vi "ADIS16448 Loop.vi"(8 "error in":errorcluster) -> ()   [LabVIEW 2025]
uses:
  <vilib>/Rock Robotics/WPI/ThirdParty/ADI/ADIS16448/Typedef/ADIS16448 Device Reference.ctl
  <vilib>/Rock Robotics/WPI/ThirdParty/ADI/ADIS16448/Typedef/ADIS16448 Hardware Configuration.ctl
  <vilib>/Rock Robotics/WPI/SPI/WPI_SPIMode.ctl
  <vilib>/Rock Robotics/SystemInterfaces/DIO/FPGA_DIOChannel.ctl
  <vilib>/Rock Robotics/SystemInterfaces/spilib/spi_bus.ctl
  <vilib>/Rock Robotics/WPI/ThirdParty/ADI/ADIS16448/Typedef/ADIS16448 Status.ctl
  <vilib>/Rock Robotics/WPI/ThirdParty/ADI/ADIS16448/Typedef/ADIS16448 Process.ctl
  <vilib>/Rock Robotics/WPI/ThirdParty/ADI/ADIS16448/Typedef/ADIS16448 Command Type.ctl
  <vilib>/Rock Robotics/SystemInterfaces/CounterEncoderSourceConvertion/FPGA_CounterEncoderSourceConvertionLVSourceType.ctl
  <vilib>/Rock Robotics/SystemInterfaces/DIO/FPGA_DIODigitalSourceChannel.ctl
  <vilib>/Rock Robotics/SystemInterfaces/AnalogTrigger/FPGA_AnalogTriggerIndex.ctl
  <vilib>/Rock Robotics/SystemInterfaces/AnalogTrigger/FPGA_AnalogTriggerOutType.ctl
  <vilib>/Rock Robotics/WPI/ThirdParty/ADI/ADIS16448/Typedef/ADIS16448 Data.ctl
  <vilib>/Rock Robotics/WPI/SPI/WPI_SPIDevRef.ctl
  <vilib>/Rock Robotics/WPI/ThirdParty/ADI/ADIS16448/Typedef/ADIS16448 Register.ctl
  <vilib>/Rock Robotics/WPI/Counter/WPI_CounterDigitalInputToDigitalSource.vi
panel:
  in  "ADIS16448DevRef":T1={"DevStatus"={"status"=FALSE, "code"=0, "source"=""}, "Hardware Config"={"SPI Clock Rate (Hz)"=1000000.0, "IMU SPI Mode (3)"=enum."Mode 3 (Clk Idle High,Sample on Trailing)", "IMU Reset Pin"=enum."SPI Port CS2", "IMU SPI Bus"=enum."SPI On-Board, CS0", "IMU Data Ready Pin"=enum."SPI Port CS1", "Stall Config"={"Pow2BytesPerRead"=255, "StallTicks"=640, "CsToSclkTicks"=5}, "IMU Status LED Pin"=enum."DIO MXP 9"}, "Calibration Complete"=refnum, "Status reference"=refnum, "Sychronous Process VI"=refnum, "Cmd FIFO"=refnum, "Source"={"DevStatus"={"status"=FALSE, "code"=0, "source"=""}, "AnalogTriggerMode?"=FALSE, "DigitalMode"={"DIO Channel"=enum."Disabled"}, "AnalogTriggerMode"={"AnalogTriggerIndex"=enum."Trig 0", "OutputType"=enum."InWindow"}}, "Data FIFO"=refnum, "IMU Status LED Pin"=enum."DIO MXP 9", "Calibration Time (ms)"=5, "Data Reference"=refnum}
  in  "Main Name":string
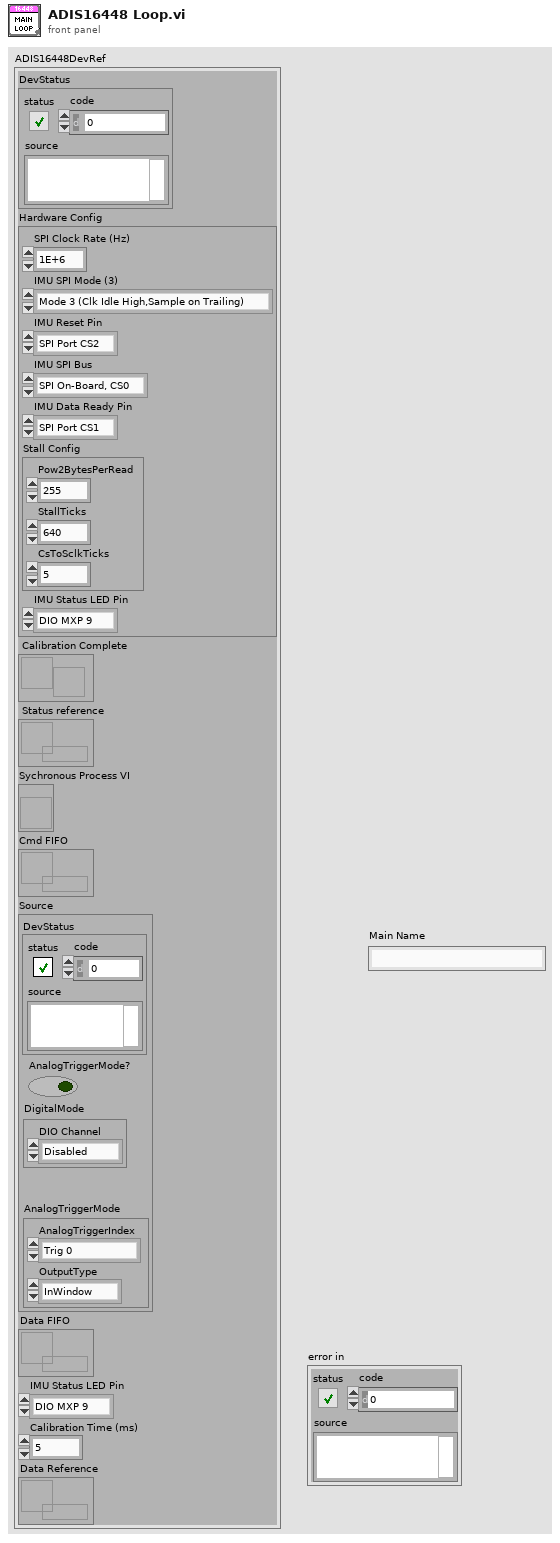
[diagram p1: front panel]
types:
  T1 = typedef "ADIS16448 Device Reference.ctl" = cluster{"DevStatus":errorcluster, "Hardware Config":T2, "Calibration Complete":refnum<notifier>, "Status reference":refnum<data-value>, "Sychronous Process VI":T6, "Cmd FIFO":refnum<k33>, "Source":T7, "Data FIFO":refnum<k33>, "IMU Status LED Pin":T4, "Calibration Time (ms)":u32, "Data Reference":refnum<data-value>}
  T2 = typedef "ADIS16448 Hardware Configuration.ctl" = cluster{"SPI Clock Rate (Hz)":dbl, "IMU SPI Mode (3)":T3, "IMU Reset Pin":T4, "IMU SPI Bus":T5, "IMU Data Ready Pin":T4, "Stall Config":cluster{"Pow2BytesPerRead":u8, "StallTicks":u16, "CsToSclkTicks":u8}, "IMU Status LED Pin":T4}
  T3 = typedef "WPI_SPIMode.ctl" = enum16{"Mode 0 (Clk Idle Low,Sample on Leading)", "Mode 1 (Clk Idle Low,Sample on Trailing)", "Mode 2 (Clk Idle High,Sample on Leading)", "Mode 3 (Clk Idle High,Sample on Trailing)"}
  T4 = typedef "FPGA_DIOChannel.ctl" = enum8{"DIO 0", "DIO 1", "DIO 2", "DIO 3", "DIO 4", "DIO 5", "DIO 6", "DIO 7", "DIO 8", "DIO 9", "DIO MXP 0", "DIO MXP 1", "DIO MXP 2", "DIO MXP 3", "DIO MXP 4", "DIO MXP 5", "DIO MXP 6", "DIO MXP 7", "DIO MXP 8", "DIO MXP 9", "DIO MXP 10", "DIO MXP 11", "DIO MXP 12", "DIO MXP 13", "DIO MXP 14", "DIO MXP 15", "SPI Port CS1", "SPI Port CS2", "SPI Port CS3", "SPI Port MISO", "SPI Port MOSI", "Invalid"}
  T5 = typedef "spi_bus.ctl" = enum16{"SPI On-Board, CS0", "SPI On-Board, CS1", "SPI On-Board, CS2", "SPI On-Board, CS3", "SPI MXP", "Invalid"}
  T6 = typedef "ADIS16448 Process.ctl" = refnum<vi>
  T7 = typedef "FPGA_CounterEncoderSourceConvertionLVSourceType.ctl" = cluster{"DevStatus":errorcluster, "AnalogTriggerMode?":bool, "DigitalMode":cluster{"DIO Channel":T8}, "AnalogTriggerMode":cluster{"AnalogTriggerIndex":T9, "OutputType":T10}}
  T8 = typedef "FPGA_DIODigitalSourceChannel.ctl" = enum8{"DIO 0", "DIO 1", "DIO 2", "DIO 3", "DIO 4", "DIO 5", "DIO 6", "DIO 7", "DIO 8", "DIO 9", "DIO MXP 0", "DIO MXP 1", "DIO MXP 2", "DIO MXP 3", "DIO MXP 4", "DIO MXP 5", "DIO MXP 6", "DIO MXP 7", "DIO MXP 8", "DIO MXP 9", "DIO MXP 10", "DIO MXP 11", "DIO MXP 12", "DIO MXP 13", "DIO MXP 14", "DIO MXP 15", "SPI Port CS1", "SPI Port CS2", "SPI Port CS3", "SPI Port MISO", "SPI Port MOSI", "Disabled"}
  T9 = typedef "FPGA_AnalogTriggerIndex.ctl" = enum8{"Trig 0", "Trig 1", "Trig 2", "Trig 3", "Trig 4", "Trig 5", "Trig 6", "Trig 7", "Invalid"}
  T10 = typedef "FPGA_AnalogTriggerOutType.ctl" = enum16{"InWindow", "TriggerState", "Rising", "Falling"}
  T11 = typedef "WPI_SPIDevRef.ctl" = cluster{"DevStatus":errorcluster, "Handle":i32, "SPI Bus":T5}
  T12 = typedef "ADIS16448 Data.ctl" = cluster{"XAngle":dbl, "YAngle":dbl, "ZAngle":dbl}
  T13 = cluster{"SPIDevRef":T11, "Data Counter":u16, "Digital Source":T7, "Bytes Per Sample":u32, "Data":T12, "ADIS16448DevRef":T1, "TimeStampPrev":u32, "Sensor to Robot Rotation":dbl[][], "AutoSPI Active?":bool, "Offsets":T12, "Data Header":u8[], "Zero Byte Count":u8, "Reset":bool}
  T14 = typedef "ADIS16448 Status.ctl" = cluster{"Calibrated?":bool, "IMU Detected?":bool}
  T15 = typedef "ADIS16448 Register.ctl" = u8
  T16 = typedef "ADIS16448 Command Type.ctl" = cluster{"Command":enum16{"None", "Reset", "Recalibrate"}, "Data":u32}
  T17 = typedef "WPI_DigitalOutputDevRef.ctl" = cluster{"DIO Channel":T4, "DevStatus":errorcluster}
  T18 = typedef "WPI_DigitalInputDevRef.ctl" = cluster{"DevStatus":errorcluster, "DIO Channel":T4}
  T19 = cluster{"Pow2BytesPerRead":u8, "StallTicks":u16, "CsToSclkTicks":u8}
  T20 = enum32{"Bad", "Idle", "Run top level", "Running"}
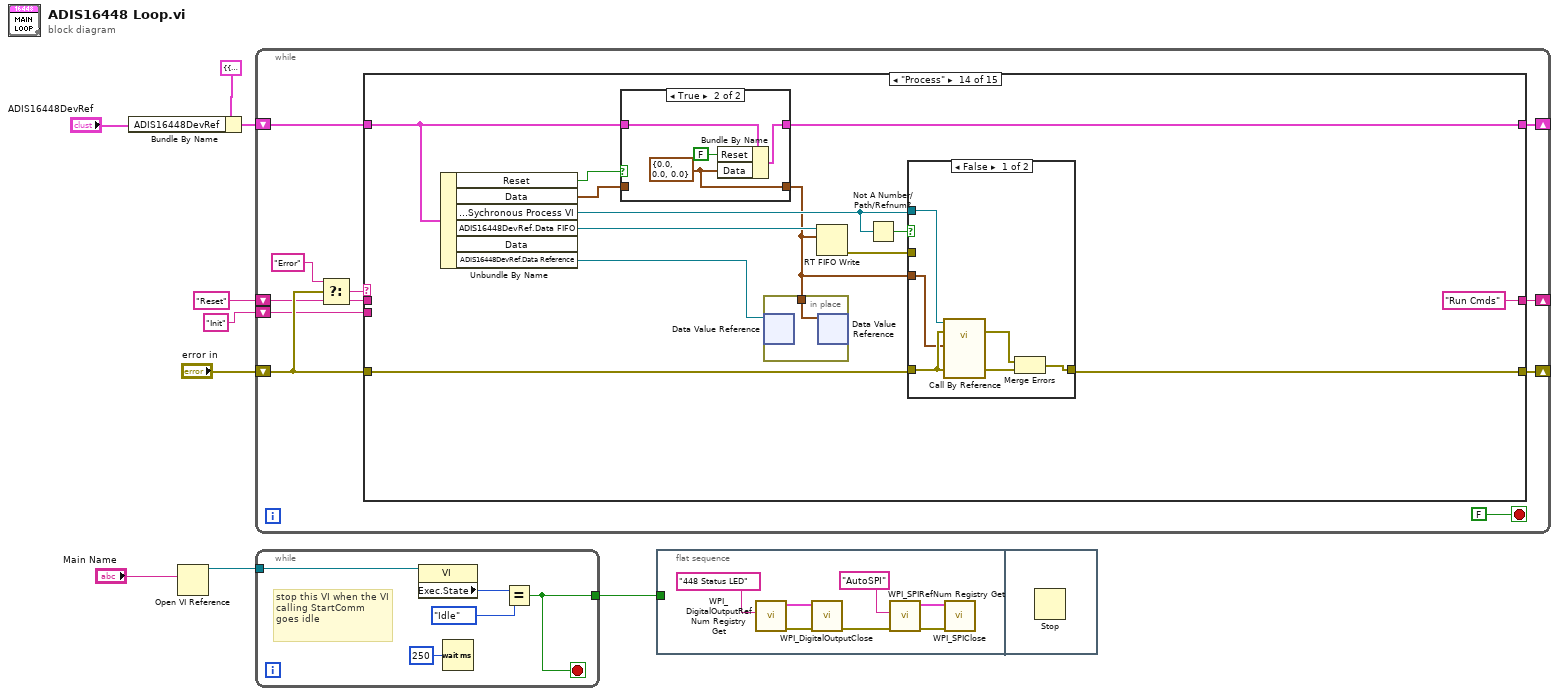
[diagram p0: block diagram]
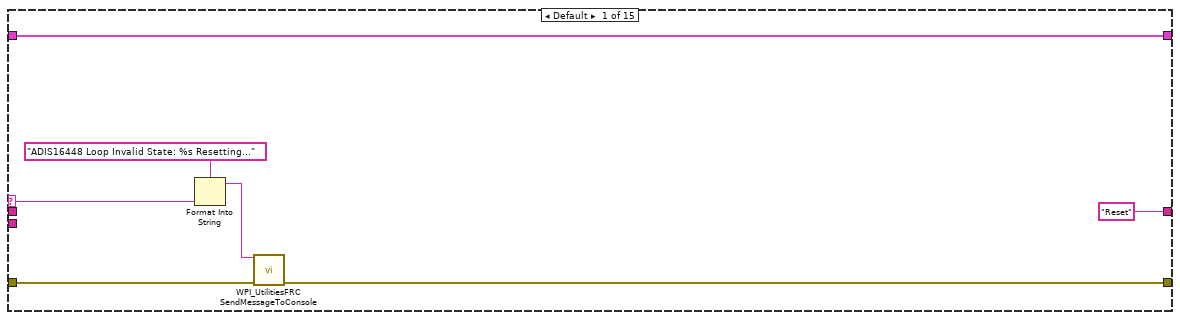
[diagram p2: hidden frame]
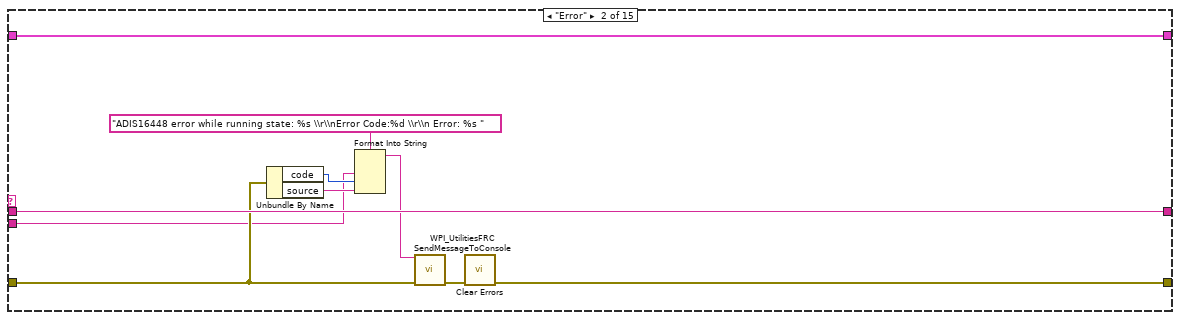
[diagram p3: hidden frame]
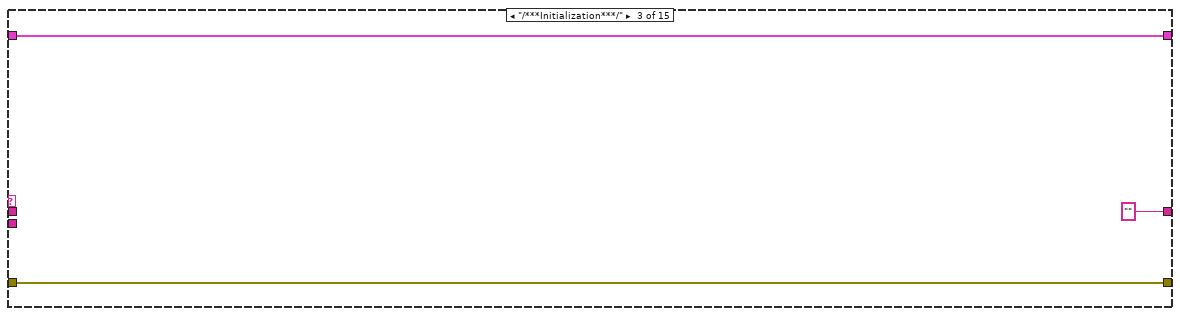
[diagram p4: hidden frame]
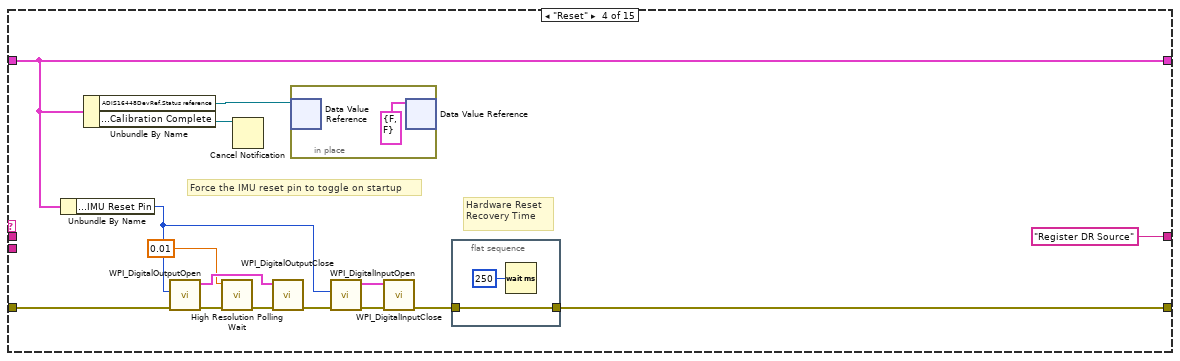
[diagram p5: hidden frame]
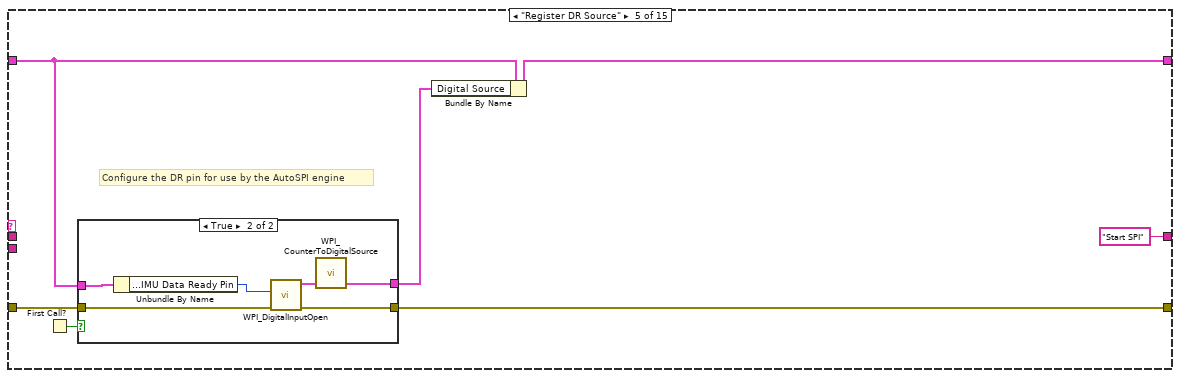
[diagram p6: hidden frame]
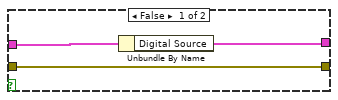
[diagram p7: hidden frame]
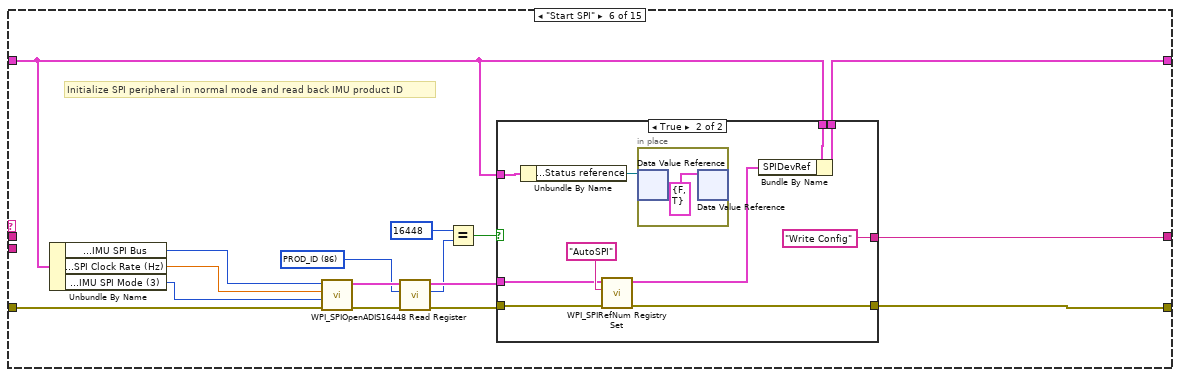
[diagram p8: hidden frame]
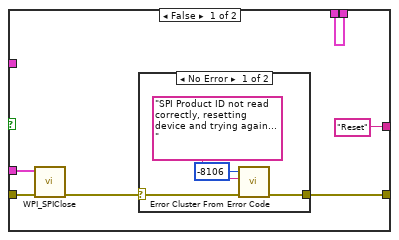
[diagram p9: hidden frame]
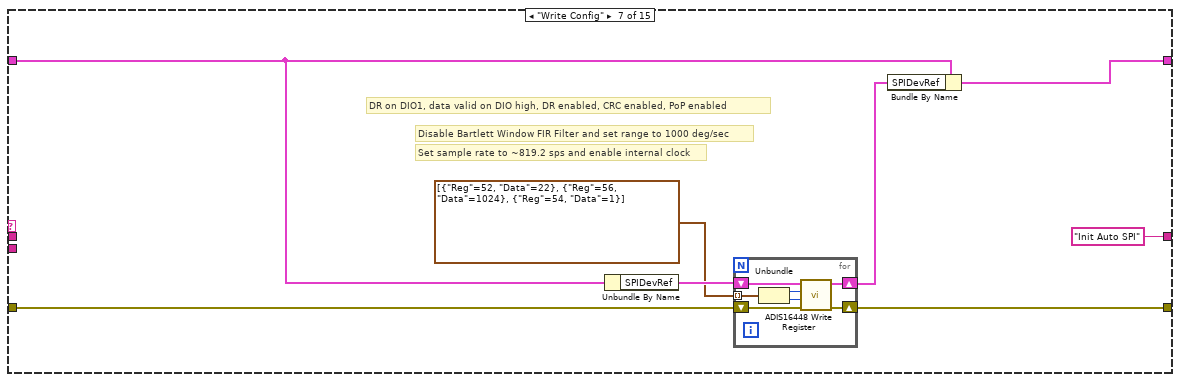
[diagram p11: hidden frame]
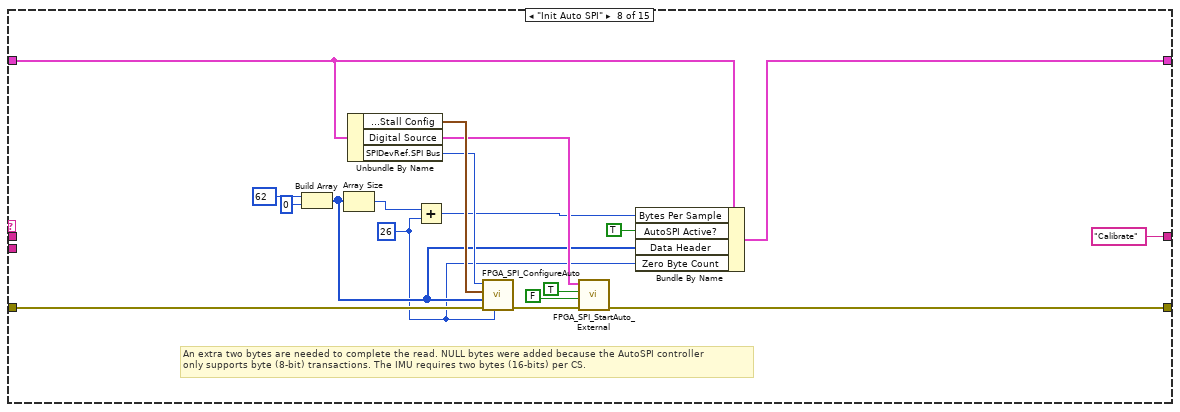
[diagram p12: hidden frame]
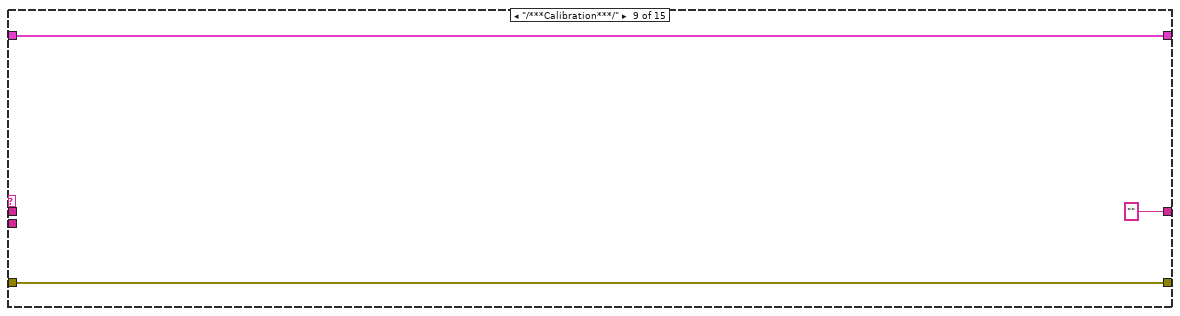
[diagram p13: hidden frame]
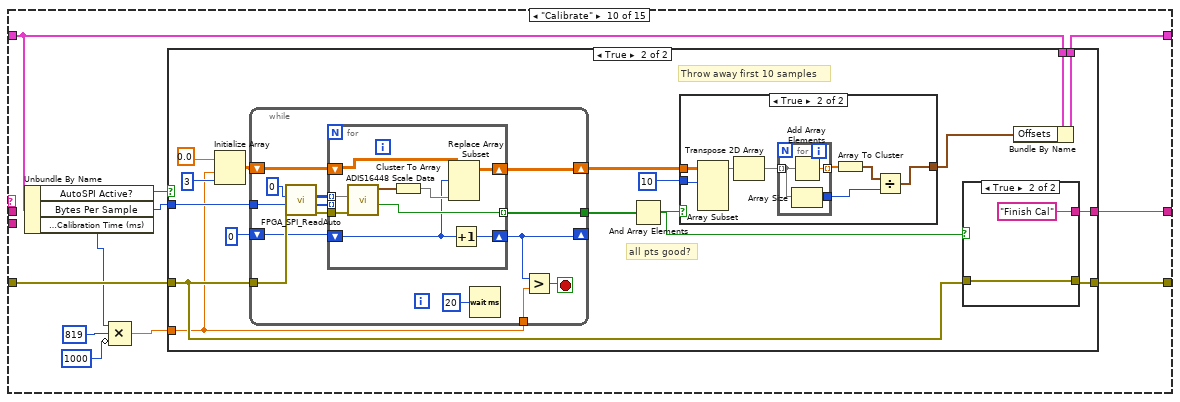
[diagram p14: hidden frame]
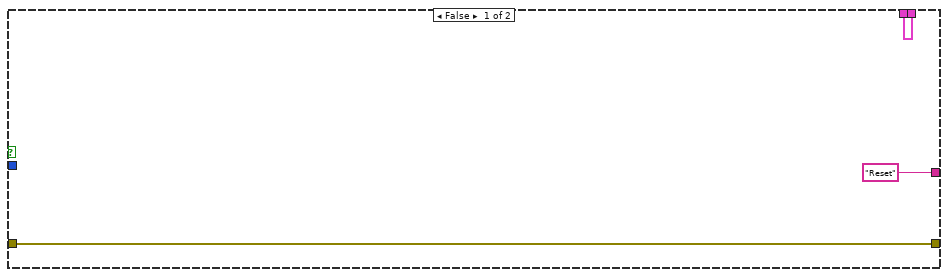
[diagram p15: hidden frame]
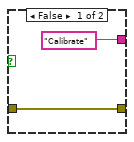
[diagram p17: hidden frame]
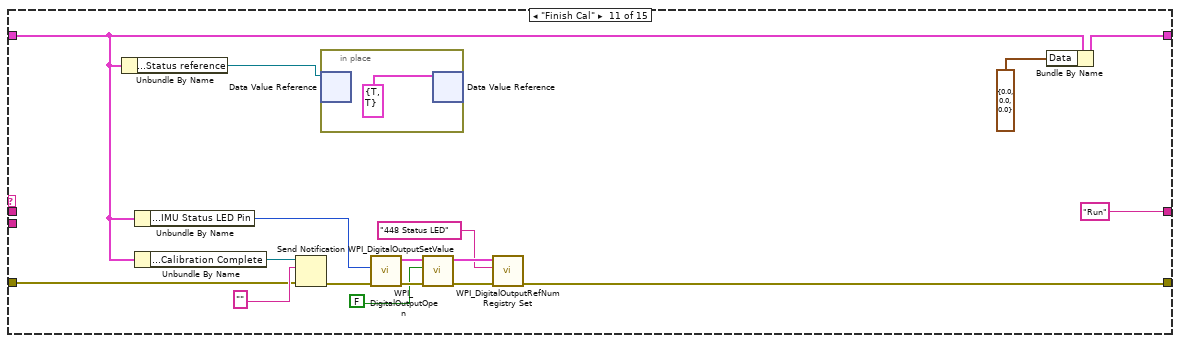
[diagram p18: hidden frame]
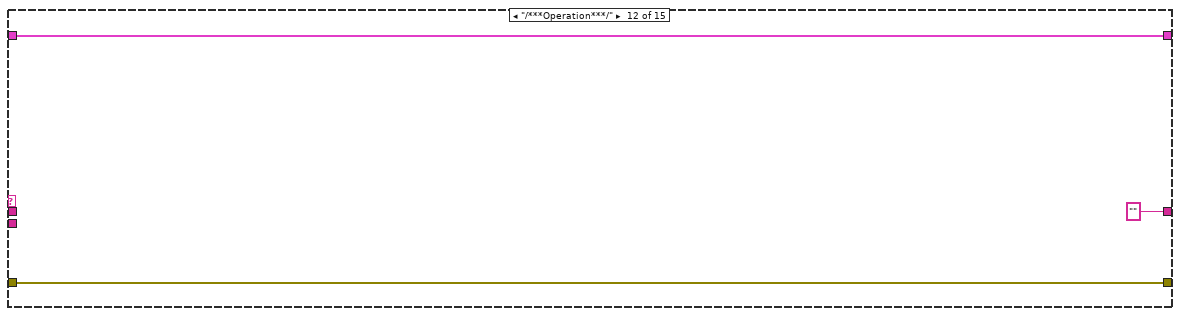
[diagram p19: hidden frame]
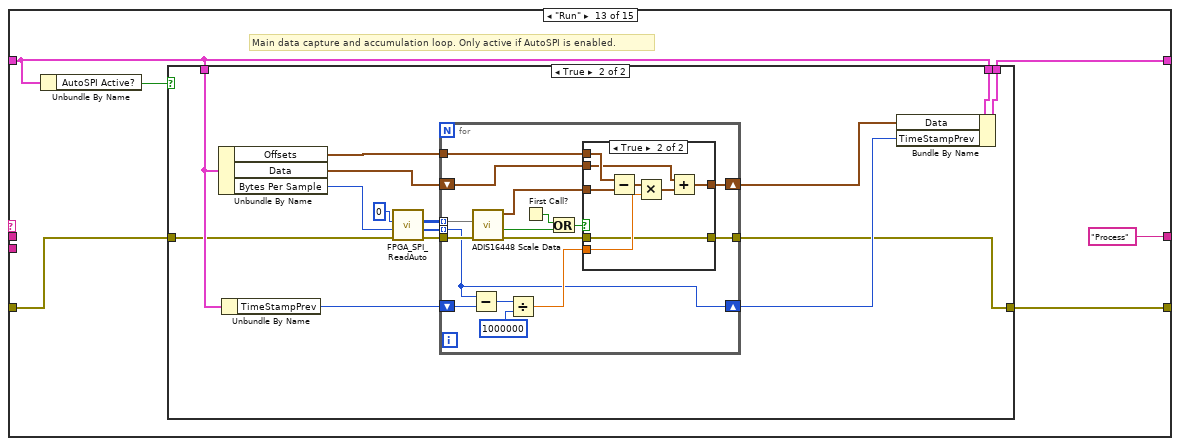
[diagram p20: hidden frame]
diagram:
  n1 = Bundle By Name(cluster=T13 {"SPIDevRef"={"DevStatus"={"status"=FALSE, "code"=0, "source"=""}, "Handle"=0, "SPI Bus"=enum."SPI On-Board, CS0"}, "Data Counter"=0, "Digital Source"={"DevStatus"={"status"=FALSE, "code"=0, "source"=""}, "AnalogTriggerMode?"=FALSE, "DigitalMode"={"DIO Channel"=enum."DIO 1"}, "AnalogTriggerMode"={"AnalogTriggerIndex"=enum."Trig 0", "OutputType"=enum."InWindow"}}, "Bytes Per Sample"=0, "Data"={"XAngle"=0.0, "YAngle"=0.0, "ZAngle"=0.0}, "ADIS16448DevRef"={"DevStatus"={"status"=FALSE, "code"=0, "source"=""}, "Hardware Config"={"SPI Clock Rate (Hz)"=1000000.0, "IMU SPI Mode (3)"=enum."Mode 3 (Clk Idle High,Sample on Trailing)", "IMU Reset Pin"=enum."SPI Port CS2", "IMU SPI Bus"=enum."SPI On-Board, CS0", "IMU Data Ready Pin"=enum."SPI Port CS1", "Stall Config"={"Pow2BytesPerRead"=255, "StallTicks"=640, "CsToSclkTicks"=5}, "IMU Status LED Pin"=enum."DIO MXP 9"}, "Calibration Complete"=refnum, "Status reference"=refnum, "Sychronous Process VI"=refnum, "Cmd FIFO"=refnum, "Source"={"DevStatus"={"status"=FALSE, "code"=0, "source"=""}, "AnalogTriggerMode?"=FALSE, "DigitalMode"={"DIO Channel"=enum."Disabled"}, "AnalogTriggerMode"={"AnalogTriggerIndex"=enum."Trig 0", "OutputType"=enum."InWindow"}}, "Data FIFO"=refnum, "IMU Status LED Pin"=enum."DIO MXP 9", "Calibration Time (ms)"=5, "Data Reference"=refnum}, "TimeStampPrev"=0, "Sensor to Robot Rotation"=[], "AutoSPI Active?"=TRUE, "Offsets"={"XAngle"=0.0, "YAngle"=0.0, "ZAngle"=0.0}, "Data Header"=[], "Zero Byte Count"=0, "Reset"=TRUE}, "ADIS16448DevRef"="ADIS16448DevRef") -> (w5:T13)
  n2 = Open VI Reference(vi path="Main Name") -> (vi reference=w8:refnum<vi>)  [unwired: 3 in, 3 out]
  n3 = while {
    shift-right: [w15] -> _
    shift-left: "Reset" -> [w12]
    shift-right: [w17] -> _
    shift-left: w5 -> [w18]
    shift-right: [w16] -> _
    shift-left: "error in" -> [w14]
    shift-left: "Init" -> [w10]
    stop <- FALSE stop-if-true
    n4 = Select(t="Error", s=w14, f=w12) -> (s? t:f=w13:string)
    n5 = case shown="\"Process\"" w13 {
      selector: w13 -> [w25 _ _ _ _ _ _ _ _ _ _ _ _ _ _]
      tunnel: w18 -> [w26 w36 w39 w40 w59 w78 w114 w139 w147 w152 w227 w236 w238 w289 w316]
      tunnel: [w26 w36 w39 w40 w63 w83 w113 w138 w147 w155 w231 w236 w241 w290 w322] -> w17
      tunnel: w14 -> [w24 w32 w38 w46 w62 w89 w117 w143 w146 w157 w228 w235 w240 w296 w324]
      tunnel: [w23 w33 w38 w53 w60 w82 w116 w127 w146 w156 w220 w235 w239 w295 w323] -> w16
      tunnel: ["Reset" w35 "" "Register DR Source" "Start SPI" w84 "Init Auto SPI" "Calibrate" "" w153 "Run" "" "Process" "Run Cmds" w314] -> w15
      tunnel: w12 -> [_ w35 _ _ _ _ _ _ _ _ _ _ _ _ _]
      tunnel: w10 -> [_ w27 _ _ _ _ _ _ _ _ _ _ _ _ _]
      frame Default {
        n6 = Format Into String(format string="ADIS16448 Loop Invalid State: %s Resetting...", w25) -> (resulting string=w22:string)  [unwired: 2 in, 1 out]
        n7 = call <vilib>:"WPI_UtilitiesFRC SendMessageToConsole.vi"("Message"=w22, "error in (no error)"=w24) -> ("error out"=w23:errorcluster)  [unwired: 13 in]
      }
      frame "Error" {
        n8 = Unbundle By Name(w32) -> ("code"=w29:i32, "source"=w28:string)
        n9 = Format Into String(format string="ADIS16448 error while running state: %s \\r\\nError Code:%d \\r\\n Error: %s ", w27, w29, w28) -> (resulting string=w31:string)  [unwired: 2 in, 1 out]
        n10 = call <vilib>:"WPI_UtilitiesFRC SendMessageToConsole.vi"("Message"=w31, "error in (no error)"=w32) -> ("error out"=w34:errorcluster)  [unwired: 13 in]
        n11 = call <vilib>:"Clear Errors.vi"("error in (no error)"=w34) -> ("error out"=w33:errorcluster)  [unwired: 5 in, 1 out]
      }
      frame "/***Initialization***/" {
      }
      frame "Reset" {
        # "Hardware Reset Recovery Time"
        # "Force the IMU reset pin to toggle on startup"
        n12 = Unbundle By Name(w40) -> ("ADIS16448DevRef.Hardware Config.IMU Reset Pin"=w42:T4)
        n13 = Unbundle By Name(w40) -> ("ADIS16448DevRef.Status reference"=w41:refnum<data-value>, "ADIS16448DevRef.Calibration Complete"=w52:refnum<notifier>)
        n14 = call <vilib>:"WPI_DigitalOutputOpen.vi"("error in (no error)"=w46, "DIO Channel"=w42) -> ("error out"=w44:errorcluster, "DigitalOutputDevRef"=w51:T17)  [unwired: 8 in]
        n15 = call <vilib>:"High Resolution Polling Wait.vi"("error in (no error)"=w44, "seconds to wait"=0.01) -> ("error out"=w45:errorcluster)  [unwired: 9 in]
        n16 = Cancel Notification(0:w52) -> ()  [unwired: 1 in, 3 out]
        n17 = call <vilib>:"WPI_DigitalOutputClose.vi"("error in (no error)"=w45, "DigitalOutputDevRef"=w51) -> ("error out"=w48:errorcluster)  [unwired: 9 in]
        n18 = in-place {
          n19 = in-place-dvr #1(w41) -> ()  [unwired: 2 out]
          n20 = in-place-dvr #1(T14 {"Calibrated?"=FALSE, "IMU Detected?"=FALSE} ("element")) -> ()  [unwired: 2 out]
        }
        n21 = call <vilib>:"WPI_DigitalInputOpen.vi"("error in (no error)"=w48, "DIO Channel"=w42) -> ("error out"=w49:errorcluster, "DigitalInputDevRef"=w50:T18)  [unwired: 8 in]
        n22 = call <vilib>:"WPI_DigitalInputClose.vi"("error in (no error)"=w49, "DigitalInputDevRef"=w50) -> ("error out"=w47:errorcluster)  [unwired: 9 in]
        n23 = flat-sequence {
          tunnel: [w57] -> w53
          tunnel: w47 -> [w57]
          frame #0 {
            n24 = Wait (ms)(milliseconds to wait=u32 250) -> ()  [unwired: 1 out]
          }
        }
      }
      frame "Register DR Source" {
        # "Configure the DR pin for use by the AutoSPI engine"
        n25 = First Call?() -> (First Call?: T/F=w58:bool)
        n26 = case shown="True" w58 {
          tunnel: w62 -> [w65 w73]
          tunnel: w59 -> [w67 w71]
          tunnel: [w66 w69] -> w61
          tunnel: [w65 w68] -> w60
          frame False {
            n27 = Unbundle By Name(w67) -> ("Digital Source"=w66:T7)
          }
          frame True {
            n28 = Unbundle By Name(w71) -> ("ADIS16448DevRef.Hardware Config.IMU Data Ready Pin"=w70:T4)
            n29 = call <vilib>:"WPI_DigitalInputOpen.vi"("error in (no error)"=w73, "DIO Channel"=w70) -> ("error out"=w68:errorcluster, "DigitalInputDevRef"=w72:T18)  [unwired: 8 in]
            n30 = call-poly <vilib>:"WPI_CounterToDigitalSource.vi"("DigitalInputDevRef"=w72) -> ("Digital Source"=w69:T7)  [unwired: 6 in]
          }
        }
        n31 = Bundle By Name(cluster=w59, "Digital Source"=w61) -> (w63:T13)
      }
      frame "Start SPI" {
        w77 = T15 86 items=["FLASH_CNT"=0, "Reserved 1"=2, "XGYRO_OUT"=4, "YGYRO_OUT"=6, "ZGYRO_OUT"=8, "XACCL_OUT"=10, "YACCL_OUT"=12, "ZACCL_OUT"=14, "XMAGN_OUT"=16, "YMAGN_OUT"=18, "ZMAGN_OUT"=20, "BARO_OUT"=22, "TEMP_OUT"=24, "XGYRO_OFF"=26, "YGYRO_OFF"=28, "ZGYRO_OFF"=30, "XACCL_OFF"=32, "YACCL_OFF"=34, "ZACCL_OFF"=36, "XMAGN_HIC"=38, "YMAGN_HIC"=40, "ZMAGN_HIC"=42, "XMAGN_SIC"=44, "YMAGN_SIC"=46, "ZMAGN_SIC"=48, "GPIO_CTRL"=50, "MSC_CTRL"=52, "SMPL_PRD"=54, "SENS_AVG"=56, "SEQ_CNT"=58, "DIAG_STAT"=60, "GLOB_CMD"=62, "ALM_MAG1"=64, "ALM_MAG2"=66, "ALM_SMPL1"=68, "ALM_SMPL2"=70, "ALM_CTRL"=72, "Reserved 2"=74, "Reserved 3"=76, "Reserved 4"=78, "Reserved 5"=80, "LOT_ID1"=82, "LOT_ID2"=84, "PROD_ID"=86, "SERIAL_NUM"=88] ("ADIS16448 Register")
        # "Initialize SPI peripheral in normal mode and read back IMU product ID"
        n32 = Unbundle By Name(w78) -> ("ADIS16448DevRef.Hardware Config.IMU SPI Bus"=w85:T5, "ADIS16448DevRef.Hardware Config.SPI Clock Rate (Hz)"=w86:dbl, "ADIS16448DevRef.Hardware Config.IMU SPI Mode (3)"=w87:T3)
        n33 = call <vilib>:"WPI_SPIOpen.vi"("error in"=w89, "Mode (3)"=w87, "Clock Rate (Hz)"=w86, "SPI Bus"=w85) -> ("error out"=w81:errorcluster, "SPIDevRef"=w80:T11)  [unwired: 6 in]
        n34 = call <vilib>:"ADIS16448 Read Register.vi"("error in (no error)"=w81, "ADIS16448 Register"=w77, "SPIDevRef in"=w80) -> ("error out"=w75:errorcluster, "Register Value"=w74:u16, "SPIDevRef out"=w76:T11)  [unwired: 6 in]
        n35 = Equal?(x=u16 16448 ("y"), y=w74) -> (x = y?=w88:bool)
        n36 = case shown="True" w88 {
          tunnel: ["Reset" "Write Config"] -> w84
          tunnel: w78 -> [w94 w109]
          tunnel: [w94 w108] -> w83
          tunnel: [w93 w103] -> w82
          tunnel: w75 -> [w92 w104]
          tunnel: w76 -> [w91 w105]
          tunnel: w78 -> [_ w102]
          frame False {
            n37 = call <vilib>:"WPI_SPIClose.vi"("error in (no error)"=w92, "SPIDevRef"=w91) -> ("error out"=w90:errorcluster)  [unwired: 9 in]
            n38 = case shown="No Error" w90 {
              selector: w90 -> [w98 w100]
              tunnel: [w99 w100] -> w93
              frame No Error {
                n39 = call <vilib>:"Error Cluster From Error Code.vi"("error in (no error)"=w98, "error message (\"\")"="SPI Product ID not read correctly, resetting device and trying again..." ("error message (\"\")"), "error code (0)"=-8106) -> ("error out"=w99:errorcluster)  [unwired: 6 in]
              }
              frame Error {
              }
            }
          }
          frame True {
            n40 = Unbundle By Name(w102) -> ("ADIS16448DevRef.Status reference"=w101:refnum<data-value>)
            n41 = call <vilib>:"WPI_SPIRefNum Registry Set.vi"("error in (no error)"=w104, "refnum name"="AutoSPI", "SPIDevRef"=w105) -> ("error out"=w103:errorcluster, "SPIDevRef"=w107:T11)  [unwired: 7 in]
            n42 = in-place {
              n43 = in-place-dvr #2(w101) -> ()  [unwired: 2 out]
              n44 = in-place-dvr #2(T14 {"Calibrated?"=FALSE, "IMU Detected?"=TRUE} ("element")) -> ()  [unwired: 2 out]
            }
            n45 = Bundle By Name(cluster=w109, "SPIDevRef"=w107) -> (w108:T13)
          }
        }
      }
      frame "Write Config" {
        # "DR on DIO1, data valid on DIO high, DR enabled, CRC enabled, PoP enabled"
        # "Set sample rate to ~819.2 sps and enable internal clock"
        # "Disable Bartlett Window FIR Filter and set range to 1000 deg/sec"
        n46 = Unbundle By Name(w114) -> ("SPIDevRef"=w118:T11)
        n47 = for {
          tunnel: cluster{"Reg":T15, "Data":u16}[] [{"Reg"=52, "Data"=22}, {"Reg"=56, "Data"=1024}, {"Reg"=54, "Data"=1}] -> [w126] mode=indexing
          shift-right: [w122] -> w116
          shift-left: w117 -> [w121]
          shift-right: [w120] -> w112
          shift-left: w118 -> [w123]
          n48 = Unbundle(w126) -> ("Reg"=w125:T15, "Data"=w124:u16)
          n49 = call <vilib>:"ADIS16448 Write Register.vi"("error in (no error)"=w121, "Data"=w124, "Register"=w125, "SPIDevRef in"=w123) -> ("error out"=w122:errorcluster, "SPIDevRef out"=w120:T11)  [unwired: 6 in]
        }
        n50 = Bundle By Name(cluster=w114, "SPIDevRef"=w112) -> (w113:T13)
      }
      frame "Init Auto SPI" {
        w128 = u8 26 ("dimension size")
        # "An extra two bytes are needed to complete the read. NULL bytes were added because the AutoSPI controller \nonly supports byte (8-bit) transactions. The IMU requires two bytes (16-bits) per CS."
        n51 = Build Array(u8 62 ("hi"), u8 0 ("element")) -> (w129:u8[])
        n52 = Array Size(array=w129) -> (size(s)=w133:i32)
        n53 = Unbundle By Name(w139) -> ("ADIS16448DevRef.Hardware Config.Stall Config"=w137:T19, "Digital Source"=w135:T7, "SPIDevRef.SPI Bus"=w134:T5)
        n54 = Add(x=w133, y=w128) -> (x+y=w130:i32)
        n55 = call <vilib>:"FPGA_SPI_ConfigureAuto.vi"("SPI Auto Zero Byte Count"=w128, "error in"=w143, "SPI Auto TX Byte Array"=w129, "Stall Config"=w137, "SPI Bus"=w134) -> ("error out"=w142:errorcluster)  [unwired: 6 in]
        n56 = call <vilib>:"FPGA_SPI_StartAuto_External.vi"("error in (no error)"=w142, "Falling Edge"=FALSE, "Rising Edge"=TRUE, "Source"=w135) -> ("error out"=w127:errorcluster)  [unwired: 7 in]
        n57 = Bundle By Name(cluster=w139, "Bytes Per Sample"=w130, "AutoSPI Active?"=TRUE, "Data Header"=w129, "Zero Byte Count"=w128) -> (w138:T13)
      }
      frame "/***Calibration***/" {
      }
      frame "Calibrate" {
        n58 = Unbundle By Name(w152) -> ("AutoSPI Active?"=w158:bool, "Bytes Per Sample"=w154:u32, "ADIS16448DevRef.Calibration Time (ms)"=w150:u32)
        n59 = Compound Arithmetic op=MULTIPLY(w150, 819, invert 1000) -> (w149:dbl)
        n60 = case shown="True" w158 {
          tunnel: [w161 w177] -> w155
          tunnel: w157 -> [w160 w165]
          tunnel: [w160 w173] -> w156
          tunnel: w152 -> [w161 w176]
          tunnel: w154 -> [_ w175]
          tunnel: ["Reset" w174] -> w153
          tunnel: w149 -> [_ w163]
          frame False {
          }
          frame True {
            # "all pts good?"
            # "Throw away first 10 samples"
            n61 = Initialize Array(0.0, w163, 3) -> (w167:dbl[][])
            n62 = while {
              tunnel: w175 -> [w187]
              tunnel: w165 -> [w186]
              tunnel: [w185] -> w172
              tunnel: w163 -> [w179]
              shift-right: [w182] -> w164
              shift-left: w167 -> [w183]
              shift-right: [w180] -> _
              shift-left: u32 0 ("Samples to Read") -> [w181]
              stop <- w178 stop-if-true
              n63 = call <vilib>:"FPGA_SPI_ReadAuto.vi"("error in (no error)"=w186, "Bytes per Sample"=w187, "Samples to Read"=u32 0) -> ("error out"=w188:errorcluster, "Timestamps"=w189:u32[], "Data"=w190:u8[][])  [unwired: 6 in]
              n64 = for {
                tunnel: w190 -> [w200] mode=indexing
                tunnel: w189 -> [_] mode=indexing
                tunnel: w188 -> [w199]
                tunnel: [w198] -> w185 mode=indexing
                shift-right: [w195] -> w182
                shift-left: w183 -> [w196]
                shift-right: [w197] -> w180
                shift-left: w181 -> [w193]
                n65 = call <vilib>:"ADIS16448 Scale Data.vi"("error in (no error)"=w199, "New Data In"=w200) -> ("Data Good?"=w198:bool, "output cluster"=w192:T12)  [unwired: 6 in, 2 out]
                n66 = Cluster To Array(cluster=w192) -> (array=w194:dbl[])
                n67 = Replace Array Subset(array=w196, new element=w194, index (row)=w193) -> (w195:dbl[][])  [unwired: 1 in]
                n68 = Increment(x=w193) -> (x+1=w197:u32)
              }
              n69 = Wait (ms)(milliseconds to wait=u32 20) -> ()  [unwired: 1 out]
              n70 = Greater?(x=w180, y=w179) -> (0:w178:bool)
            }
            n71 = And Array Elements(Boolean array=w172) -> (logical AND=w170:bool)
            n72 = case shown="True" w170 {
              tunnel: 10 -> [_ w207]
              tunnel: w164 -> [_ w208]
              tunnel: [_ w203] -> w162
              frame False {
              }
              frame True {
                n73 = Array Subset(array=w208, index (row)=w207) -> (w206:dbl[][])  [unwired: 3 in]
                n74 = Transpose 2D Array(2D array=w206) -> (transposed array=w202:dbl[][])
                n75 = for {
                  tunnel: w202 -> [w210] mode=indexing
                  tunnel: [w211] -> w205 mode=indexing
                  tunnel: [w209] -> w201
                  n76 = Add Array Elements(numeric array=w210) -> (sum=w211:dbl)
                  n77 = Array Size(array=w210) -> (size(s)=w209:i32)
                }
                n78 = Array To Cluster(array=w205) -> (cluster=w204:cluster{"[0]":dbl, "[1]":dbl, "[2]":dbl})
                n79 = Divide(x=w204, y=w201) -> (x/y=w203:cluster{"[0]":dbl, "[1]":dbl, "[2]":dbl})
              }
            }
            n80 = case shown="True" w170 {
              tunnel: ["Calibrate" "Finish Cal"] -> w174
              tunnel: [w212 w214] -> w173
              tunnel: w165 -> [w212 w214]
              frame False {
              }
              frame True {
              }
            }
            n81 = Bundle By Name(cluster=w176, "Offsets"=w162) -> (w177:T13)
          }
        }
      }
      frame "Finish Cal" {
        n82 = Unbundle By Name(w227) -> ("ADIS16448DevRef.Status reference"=w217:refnum<data-value>)
        n83 = Unbundle By Name(w227) -> ("ADIS16448DevRef.Hardware Config.IMU Status LED Pin"=w218:T4)
        n84 = Unbundle By Name(w227) -> ("ADIS16448DevRef.Calibration Complete"=w230:refnum<notifier>)
        n85 = Send Notification(notification="", notifier=w230, error in (no error)=w228) -> (error out=w221:errorcluster)  [unwired: 1 out]
        n86 = in-place {
          n87 = in-place-dvr #3(w217) -> ()  [unwired: 2 out]
          n88 = in-place-dvr #3(T14 {"Calibrated?"=TRUE, "IMU Detected?"=TRUE} ("element")) -> ()  [unwired: 2 out]
        }
        n89 = call <vilib>:"WPI_DigitalOutputOpen.vi"("error in (no error)"=w221, "DIO Channel"=w218) -> ("error out"=w226:errorcluster, "DigitalOutputDevRef"=w225:T17)  [unwired: 8 in]
        n90 = call <vilib>:"WPI_DigitalOutputSetValue.vi"("error in (no error)"=w226, "Value"=FALSE, "DigitalOutputDevRef"=w225) -> ("error out"=w224:errorcluster, "DigitalOutputDevRef"=w223:T17)  [unwired: 7 in]
        n91 = call <vilib>:"WPI_DigitalOutputRefNum Registry Set.vi"("error in (no error)"=w224, "refnum name"="448 Status LED", "DigitalOutputDevRef"=w223) -> ("error out"=w220:errorcluster)  [unwired: 7 in, 1 out]
        n92 = Bundle By Name(cluster=w227, "Data"=T12 {"XAngle"=0.0, "YAngle"=0.0, "ZAngle"=0.0}) -> (w231:T13)
      }
      frame "/***Operation***/" {
      }
      frame "Run" {
        # "Main data capture and accumulation loop. Only active if AutoSPI is enabled."
        n93 = Unbundle By Name(w238) -> ("AutoSPI Active?"=w237:bool)
        n94 = case shown="True" w237 {
          tunnel: [w244 w259] -> w241
          tunnel: w240 -> [w243 w249]
          tunnel: [w243 w246] -> w239
          tunnel: w238 -> [w244 w253]
          tunnel: w238 -> [_ w250]
          frame False {
          }
          frame True {
            n95 = Unbundle By Name(w250) -> ("Offsets"=w247:T12, "Data"=w254:T12, "Bytes Per Sample"=w258:u32)
            n96 = Unbundle By Name(w250) -> ("TimeStampPrev"=w252:u32)
            n97 = call <vilib>:"FPGA_SPI_ReadAuto.vi"("error in (no error)"=w249, "Bytes per Sample"=w258, "Samples to Read"=u32 0) -> ("error out"=w248:errorcluster, "Timestamps"=w255:u32[], "Data"=w256:u8[][])  [unwired: 6 in]
            n98 = for {
              tunnel: w256 -> [w274] mode=indexing
              tunnel: w255 -> [w261] mode=indexing
              shift-right: [w268] -> w245
              shift-left: w254 -> [w267]
              shift-right: [w261] -> w251
              shift-left: w252 -> [w275]
              tunnel: w248 -> [w273]
              tunnel: w247 -> [w272]
              tunnel: [w265] -> w246
              n99 = Subtract(x=w261, y=w275) -> (x-y=w271:u32)
              n100 = call <vilib>:"ADIS16448 Scale Data.vi"("error in (no error)"=w273, "New Data In"=w274) -> ("error out"=w266:errorcluster, "Data Good?"=w263:bool, "output cluster"=w260:T12)  [unwired: 6 in, 1 out]
              n101 = Divide(x=w271, y=u32 1000000) -> (x/y=w269:dbl)
              n102 = First Call?() -> (First Call?: T/F=w262:bool)
              n103 = Or(x=w262, y=w263) -> (x .or. y?=w264:bool)
              n104 = case shown="True" w264 {
                tunnel: w272 -> [_ w285]
                tunnel: w269 -> [_ w283]
                tunnel: [w277 w282] -> w268
                tunnel: w267 -> [w277 w280]
                tunnel: w266 -> [w276 w279]
                tunnel: [w276 w279] -> w265
                tunnel: w260 -> [_ w278]
                frame False {
                }
                frame True {
                  n105 = Subtract(x=w285, y=w278) -> (x-y=w284:T12)
                  n106 = Multiply(x=w284, y=w283) -> (x*y=w281:T12)
                  n107 = Add(x=w280, y=w281) -> (x+y=w282:T12)
                }
              }
            }
            n108 = Bundle By Name(cluster=w253, "Data"=w245, "TimeStampPrev"=w251) -> (w259:T13)
          }
        }
      }
      frame "Process" {
        n109 = Unbundle By Name(w289) -> ("Reset"=w288:bool, "Data"=w286:T12, "ADIS16448DevRef.Sychronous Process VI"=w293:T6, "ADIS16448DevRef.Data FIFO"=w297:refnum<k33>, "ADIS16448DevRef.Data Reference"=w292:refnum<data-value>)  [unwired: 1 out]
        n110 = case shown="True" w288 {
          tunnel: [w299 w304] -> w290
          tunnel: w289 -> [w299 w303]
          tunnel: [w300 w302] -> w287
          tunnel: w286 -> [w300 _]
          frame False {
          }
          frame True {
            w302 = T12 {"XAngle"=0.0, "YAngle"=0.0, "ZAngle"=0.0} ("Data")
            n111 = Bundle By Name(cluster=w303, "Reset"=FALSE, "Data"=w302) -> (w304:T13)
          }
        }
        n112 = in-place {
          in-place-border: w287 -> [w305]
          n113 = in-place-dvr #4(w292) -> ()  [unwired: 2 out]
          n114 = in-place-dvr #4(w305) -> ()  [unwired: 2 out]
        }
        n115 = RT FIFO Write(0:w297, 1:w287) -> (11:w291:errorcluster)  [unwired: 3 in, 3 out]
        n116 = Not A Number/Path/Refnum?(number/path/refnum=w293) -> (NaN/Path/Refnum?=w294:bool)
        n117 = case shown="False" w294 {
          tunnel: w296 -> [w308 w312]
          tunnel: w287 -> [w306 _]
          tunnel: [w311 w312] -> w295
          tunnel: w293 -> [w307 _]
          tunnel: w291 -> [_ _]
          frame False {
            n118 = call-by-ref "?"(reference=w307, error in=w308, 8:"error in (no error)"=w308, "element"=w306) -> (error out=w309:errorcluster, 0:"error out"=w310:errorcluster)  [unwired: 9 in, 1 out]
            n119 = Merge Errors(w309, w310) -> (w311:errorcluster)
          }
          frame True {
          }
        }
      }
      frame "Run Cmds" {
        # "If you wan to allow API VIs to impace the state machine, add a command"
        n120 = Unbundle By Name(w316) -> ("ADIS16448DevRef.Cmd FIFO"=w325:refnum<k33>)
        n121 = Unbundle By Name(w316) -> ("ADIS16448DevRef.Status reference"=w320:refnum<data-value>, "ADIS16448DevRef.Calibration Complete"=w321:refnum<notifier>)
        n122 = RT FIFO Read(0:w325, 1:T16 {"Command"=enum."None", "Data"=0} ("element")) -> (8:w319:refnum<k33>, 9:w318:T16)  [unwired: 2 in, 3 out]
        n123 = Unbundle(w318) -> ("Command"=w315:enum16{"None", "Reset", "Recalibrate"}, "Data"=w317:u32)
        n124 = case shown="\"Recalibrate\"" w315 {
          tunnel: w316 -> [w328 w334 w338]
          tunnel: w324 -> [w329 w333 w339]
          tunnel: [w329 w333 w339] -> w323
          tunnel: [w328 w332 w337] -> w322
          tunnel: w321 -> [_ _ _]
          tunnel: w320 -> [_ _ _]
          tunnel: w319 -> [_ _ _]
          tunnel: w317 -> [_ _ w336]
          tunnel: w316 -> [_ _ _]
          tunnel: ["Run" "Run" "Calibrate"] -> w314
          frame "None", Default {
          }
          frame "Reset" {
            n125 = Bundle By Name(cluster=w334, "Reset"=TRUE) -> (w332:T13)
          }
          frame "Recalibrate" {
            n126 = Bundle By Name(cluster=w338, "ADIS16448DevRef.Calibration Time (ms)"=w336, "Reset"=TRUE) -> (w337:T13)
          }
        }
        n127 = Wait (ms)(milliseconds to wait=u32 20) -> ()  [unwired: 1 out]
      }
    }
  }
  n128 = while {
    tunnel: w8 -> [w342]
    tunnel: [w341] -> w2
    stop <- w341 stop-if-true
    # "stop this VI when the VI calling StartComm goes idle"
    n129 = property class="VI"(reference=w342) -> ("Exec.State"=w344:T20)  [unwired: 1 in, 2 out]
    n130 = Wait (ms)(milliseconds to wait=u32 250) -> ()  [unwired: 1 out]
    n131 = Equal?(x=w344, y=T20."Idle" ("Execution:State")) -> (x = y?=w341:bool)
  }
  n132 = flat-sequence {
    tunnel: w2 -> [_]
    frame #0 {
      n133 = call <vilib>:"WPI_DigitalOutputRefNum Registry Get.vi"("refnum name"="448 Status LED") -> ("error out"=w351:errorcluster, "DigitalOutputDevRef"=w350:T17)  [unwired: 9 in]
      n134 = call <vilib>:"WPI_DigitalOutputClose.vi"("error in (no error)"=w351, "DigitalOutputDevRef"=w350) -> ("error out"=w346:errorcluster)  [unwired: 9 in]
      n135 = call <vilib>:"WPI_SPIRefNum Registry Get.vi"("error in (no error)"=w346, "refnum name"="AutoSPI") -> ("error out"=w348:errorcluster, "SPIDevRef"=w347:T11)  [unwired: 8 in]
      n136 = call <vilib>:"WPI_SPIClose.vi"("error in (no error)"=w348, "SPIDevRef"=w347) -> ()  [unwired: 9 in, 1 out]
    }
    frame #1 {
      n137 = Stop() -> ()  [unwired: 1 in]
    }
  }
